vi "02_DSP_zero_cross_detektor_trochu_lepe.vi"() -> ()   [LabVIEW 2019]
uses:
  <vilib>/Analysis/baseanly.llb/Mean (DBL).vi
  <vilib>/measure/NI_MABase.lvlib
  <vilib>/Analysis/NI_AALBase.lvlib
panel:
  in  "Cas necitlivosti (s)":dbl=0.005
  out "Median frekvence (Hz)":dbl=10.001000100010002 format="%0.2f"
  out "Prumerna frekvence (Hz)":dbl=10.009034438693293 format="%0.2f"
  out "Frekvence signalu (Hz)":dbl[](array[numeric])=[10.1010101010101, 9.615384615384617, 10.416666666666664, 9.708737864077671, 9.900990099009903, 10.204081632653052, 9.708737864077671, 10.41666666666667]
  out "Perioda signalu (s)":dbl[](array[numeric])=[0.099, 0.10399999999999998, 0.09600000000000002, 0.103, 0.10099999999999998, 0.09800000000000009, 0.103, 0.09599999999999997]
  out "Pole casu pruchodu nulou":dbl[](array[numeric])=[0.0485, 0.098, 0.15, 0.198, 0.2495, 0.3, 0.34900000000000003, 0.4005, 0.4485]
  out "dt (s)":dbl=0.0005
  out "Vzorkovaci Frekvence (N)":dbl=2000.0
  out "1_XY Graph":cluster{dbl[], dbl[]}[](graph)=[{array[1000 elements], array[1000 elements]}, {[0.0485, 0.098, 0.15, 0.198, 0.2495, 0.3, 0.34900000000000003, 0.4005, 0.4485], [-0.01720993872174592, 0.1969140655374353, -0.5700493875993211, 0.05445077749840377, -0.6216968862176513, 0.38013050529623005, -0.16331188826766108, 0.9406239679402187, -0.08490239756225282]}]
  in  "Amplituda sumu":dbl=1.0 format="%.2p"
  in  "Info o vzorkovani":T1={"Vzorkovaci frekvence"=2000.0, "Pocet vzorku v okne"=1000.0} {"Vzorkovaci frekvence" format="%.2p"}
  in  "Faze":dbl format="%.2p"
  in  "Amplituda":dbl=10.0 format="%0.2p"
  in  "Frekvence":dbl=10.0 format="%0.2p"
  # "GENEROVANI SIGNALU"
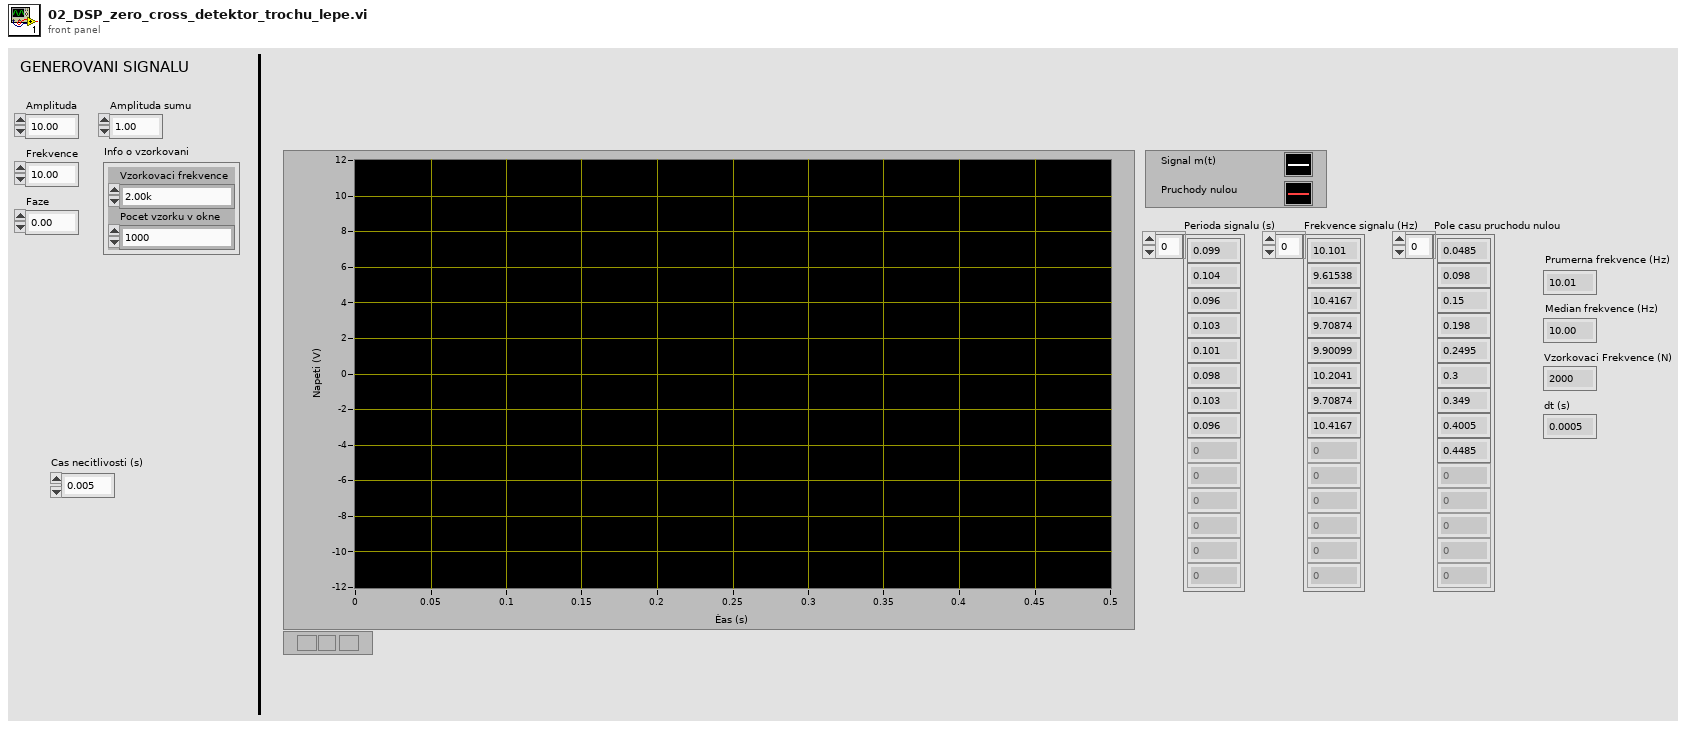
[diagram p1: front panel]
types:
  T1 = cluster{"Vzorkovaci frekvence":dbl, "Pocet vzorku v okne":dbl}
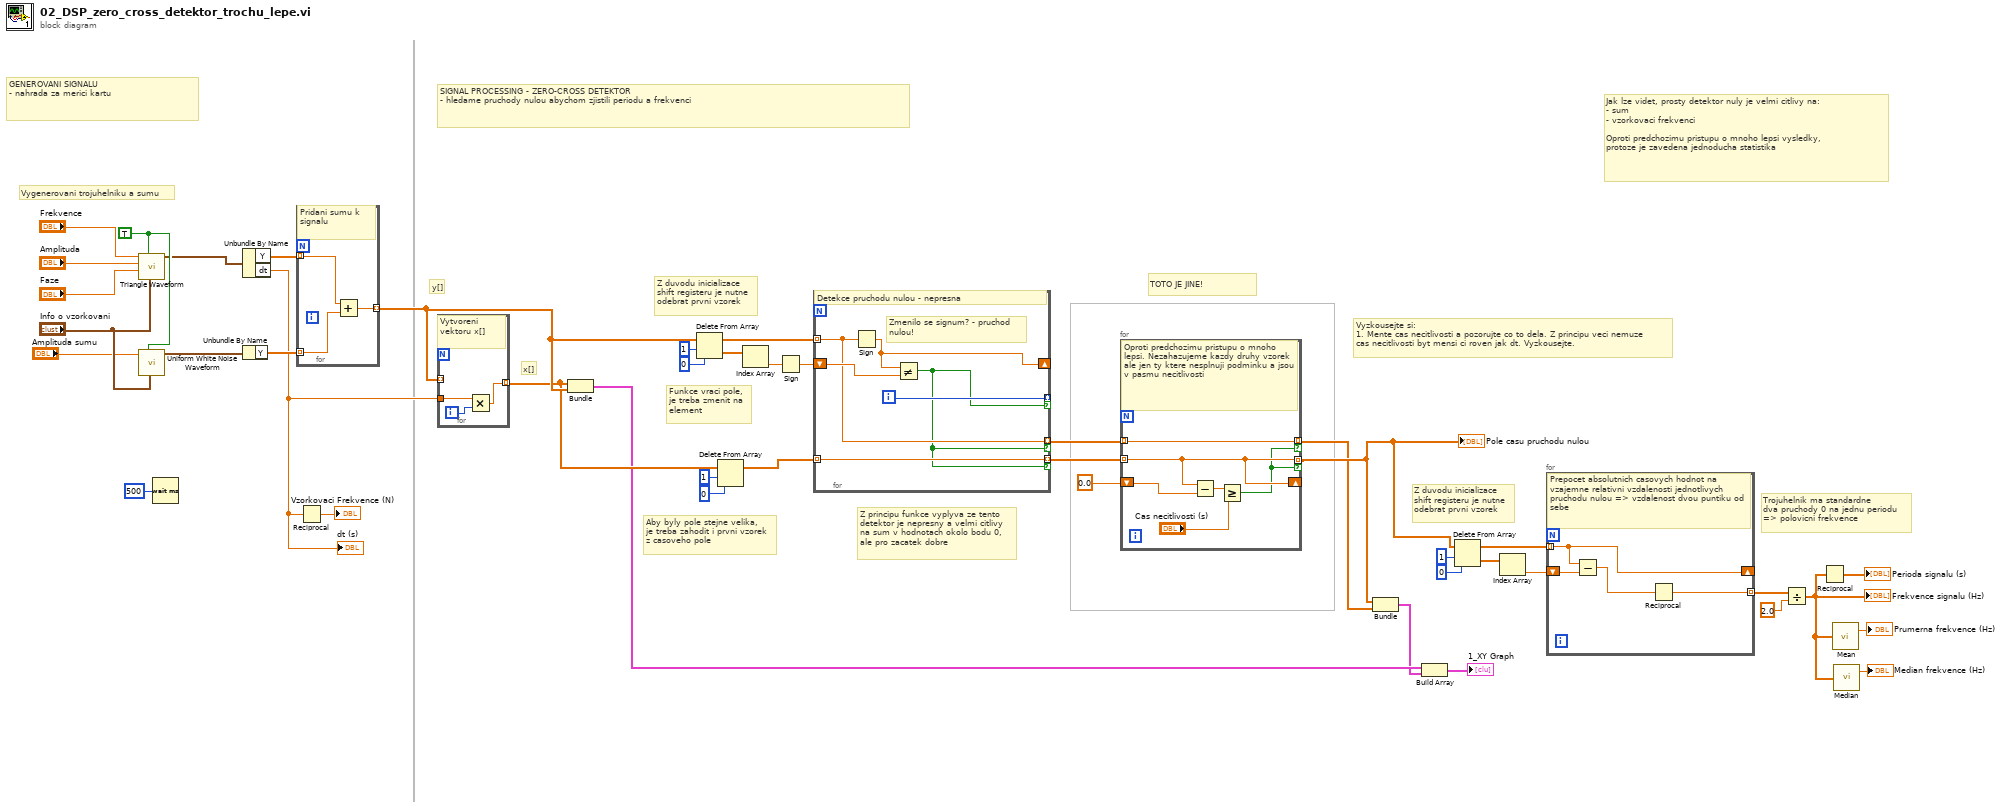
[diagram p0: block diagram]
diagram:
  w38 = TRUE ("reset signal")
  # "TOTO JE JINE!"
  # "x[]"
  # "y[]"
  # "Vyzkousejte si:\n1. Mente cas necitlivosti a pozorujte co to dela. Z principu veci nemuze \ncas necitlivosti byt mensi ci roven jak dt. Vyzkousejte."
  # "Jak lze videt, prosty detektor nuly je velmi citlivy na:\n- sum\n- vzorkovaci frekvenci\n\nOproti predchozimu pristupu o mnoho lepsi vysledky,\nprotoze je zavedena jednoducha statistika"
  # "SIGNAL PROCESSING - ZERO-CROSS DETEKTOR\n- hledame pruchody nulou abychom zjistili periodu a frekvenci"
  # "GENEROVANI SIGNALU\n- nahrada za merici kartu"
  # "Trojuhelnik ma standardne \ndva pruchody 0 na jednu periodu\n=> polovicni frekvence"
  # "Z duvodu inicializace\nshift registeru je nutne\nodebrat prvni vzorek"
  # "Z principu funkce vyplyva ze tento\ndetektor je nepresny a velmi citlivy \nna sum v hodnotach okolo bodu 0,\nale pro zacatek dobre"
  # "Aby byly pole stejne velika,\nje treba zahodit i prvni vzorek\nz casoveho pole"
  # "Funkce vraci pole,\nje treba zmenit na \nelement"
  # "Z duvodu inicializace\nshift registeru je nutne\nodebrat prvni vzorek"
  # "Vygenerovani trojuhelniku a sumu"
  n1 = call <vilib>:"Triangle Waveform.vi"("sampling info"="Info o vzorkovani", "reset signal"=w38, "phase"="Faze", "amplitude"="Amplituda", "frequency"="Frekvence") -> ("signal out"=w34:waveform(dbl))  [unwired: 5 in, 1 out]
  n2 = call <vilib>:"Uniform White Noise Waveform.vi"("sampling info"="Info o vzorkovani", "reset signal"=w38, "amplitude"="Amplituda sumu") -> ("signal out"=w37:waveform(dbl))  [unwired: 7 in, 1 out]
  n3 = Wait (ms)(milliseconds to wait=u32 500) -> ()  [unwired: 1 out]
  n4 = Unbundle By Name(w34) -> ("Y"=w36:dbl[], "dt"=w33:dbl)
  "dt (s)" <- w33
  n5 = Unbundle By Name(w37) -> ("Y"=w35:dbl[])
  n6 = for {
    tunnel: w36 -> [w45] mode=indexing
    tunnel: w35 -> [w46] mode=indexing
    tunnel: [w44] -> w31 mode=indexing
    # "Pridani sumu k signalu"
    n7 = Add(x=w45, y=w46) -> (x+y=w44:dbl)
  }
  n8 = Reciprocal(x=w33) -> (1/x=→"Vzorkovaci Frekvence (N)":dbl)
  n9 = for {
    tunnel: w31 -> [_] mode=indexing
    tunnel: w33 -> [w48]
    tunnel: [w47] -> w23 mode=indexing
    i -> [w49]
    # "Vytvoreni vektoru x[]"
    n10 = Multiply(x=w48, y=w49) -> (x*y=w47:dbl)
  }
  n11 = Bundle(w23, w31) -> (w17:cluster{dbl[], dbl[]})  [unwired: 1 in]
  n12 = Delete From Array(array=w31, length=1, index=0) -> (deleted portion=w27:dbl[], array with subset deleted=w30:dbl[])
  n13 = Delete From Array(array=w23, length=1, index=0) -> (array with subset deleted=w24:dbl[])  [unwired: 1 out]
  n14 = Index Array(array=w27) -> (element=w14:dbl)  [unwired: 1 in]
  n15 = Sign(1:w14) -> (0:w13:dbl)
  n16 = for {
    tunnel: w30 -> [w51] mode=indexing
    shift-right: [w55] -> _
    shift-left: w13 -> [w54]
    tunnel: [w53] -> _ mode=indexing if=w50
    tunnel: w24 -> [w52] mode=indexing
    tunnel: [w52] -> w6 mode=indexing if=w50
    tunnel: [w51] -> w3 mode=indexing if=w50
    i -> [w53]
    # "Zmenilo se signum? - pruchod\nnulou!"
    # "Detekce pruchodu nulou - nepresna"
    n17 = Sign(1:w51) -> (0:w55:dbl)
    n18 = Not Equal?(x=w55, y=w54) -> (x != y?=w50:bool)
  }
  n19 = for {
    tunnel: w6 -> [w58] mode=indexing
    shift-right: [w58] -> _
    shift-left: 0.0 -> [w59]
    tunnel: [w58] -> w4 mode=indexing if=w56
    tunnel: w3 -> [w57] mode=indexing
    tunnel: [w57] -> w2 mode=indexing if=w56
    # "Oproti predchozimu pristupu o mnoho lepsi. Nezahazujeme kazdy druhy vzorek ale jen ty ktere nesplnuji podminku a jsou v pasmu necitlivosti"
    n20 = Subtract(x=w58, y=w59) -> (x-y=w61:dbl)
    n21 = Greater Or Equal?(x=w61, y="Cas necitlivosti (s)") -> (x >= y?=w56:bool)
  }
  "Pole casu pruchodu nulou" <- w4
  n22 = Bundle(w4, w2) -> (w16:cluster{dbl[], dbl[]})  [unwired: 1 in]
  n23 = Build Array(w17, w16) -> (→"1_XY Graph":cluster{dbl[], dbl[]}[])
  n24 = Delete From Array(array=w4, length=1, index=0) -> (deleted portion=w22:dbl[], array with subset deleted=w19:dbl[])
  n25 = Index Array(array=w22) -> (element=w18:dbl)  [unwired: 1 in]
  n26 = for {
    tunnel: w19 -> [w65] mode=indexing
    shift-right: [w65] -> _
    shift-left: w18 -> [w64]
    tunnel: [w62] -> w12 mode=indexing
    # "Prepocet absolutnich casovych hodnot na vzajemne relativni vzdalenosti jednotlivych pruchodu nulou => vzdalenost dvou puntiku od sebe"
    n27 = Subtract(x=w65, y=w64) -> (x-y=w63:dbl)
    n28 = Reciprocal(x=w63) -> (1/x=w62:dbl)
  }
  n29 = Divide(x=w12, y=2.0) -> (x/y=w9:dbl[])
  "Frekvence signalu (Hz)" <- w9
  n30 = Reciprocal(x=w9) -> (1/x=→"Perioda signalu (s)":dbl[])
  n31 = call-poly <vilib>:"Mean.vi"("X"=w9) -> ("mean"=→"Prumerna frekvence (Hz)":dbl)  [unwired: 1 out]
  n32 = call <vilib>:"Median.vi"("X"=w9) -> ("median"=→"Median frekvence (Hz)":dbl)  [unwired: 1 out]
